vi "READ Falcon500 values.vi"(0 "PhoenixMotorControlDevRef":T1, 1 "refnum name":string, 3 "error in (no error)":errorcluster) -> (6 "PhoenixMotorControlDevRef 2":T1={"DeviceStatus"={"status"=FALSE, "code"=0, "source"=""}, "Type"=enum."PWM", "PWM"={"PWM Channel"=enum."Invalid", "DeadBand"={"Name"="", "maxPositivePwm"=0, "minPositivePwm"=0, "centerPwm"=0, "maxNegativePwm"=0, "minNegativePwm"=0, "angularRange"=0}}, "CAN"={"Device Number"=0, "SetOutput VI Ref"=variant(enum8{"Percent VBus", "Current", "Speed", "Position", "Voltage"} enum."Percent VBus"), "GetOutput VI Ref"=variant(refnum<k1> refnum), "Enable VI Ref"=variant(dbl 12.0), "Disable VI Ref"=variant(enum8{"Percent VBus", "Speed", "Position", "Slave", "Unchanged / Invalid", "Voltage Compensation", "Current", "Motion Profile"} enum."Percent VBus"), "Data"=variant}, "Invert"=FALSE, "DIO PWM"={"PWM \"Enable\" Channel"=enum."Invalid", "DIOChannel"=enum."Invalid", "PWM Rate"=0.0}}, 9 "error out":errorcluster)   [LabVIEW 2020]
uses:
  <vilib>/Rock Robotics/WPI/MotorControl/WPI_MotorControlDeviceRef.ctl
  <vilib>/Rock Robotics/WPI/MotorControl/WPI_MotorControlType.ctl
  <vilib>/Rock Robotics/SystemInterfaces/DIO/FPGA_DIOPWMChannel.ctl
  <vilib>/Rock Robotics/WPI/PWM/WPI_PWMDeadband.ctl
  <vilib>/Rock Robotics/SystemInterfaces/DIO/FPGA_DIOChannel.ctl
  <vilib>/Rock Robotics/WPI/ThirdParty/Phoenix-LabVIEW/Motor Controller/Get/CTRE_Phoenix_MotorController_GetVoltage.vi
  <vilib>/Rock Robotics/Network Tables/NT Write Number.vi
  <vilib>/Rock Robotics/WPI/ThirdParty/Phoenix-LabVIEW/Motor Controller/Get/CTRE_Phoenix_MotorController_GetSupplyAndStatorCurrent_Enhanced.vi
  <vilib>/Rock Robotics/WPI/ThirdParty/Phoenix-LabVIEW/Motor Controller/Get/CTRE_Phoenix_MotorController_GetSelectedSensorData.vi
  <vilib>/Rock Robotics/WPI/ThirdParty/Phoenix-LabVIEW/Motor Controller/Get/CTRE_Phoenix_MotorController_IntegratedSensorData_TalonFX.vi
  <vilib>/Rock Robotics/WPI/ThirdParty/Phoenix-LabVIEW/Motor Controller/Get/CTRE_Phoenix_MotorController_GetTemperature.vi
  <vilib>/Rock Robotics/WPI/ThirdParty/Phoenix-LabVIEW/Motor Controller/Get/CTRE_Phoenix_MotorController_GetLimitSwitchStates.vi
  <vilib>/Rock Robotics/Network Tables/NT Write Boolean.vi
panel:
  in  "ticks per rev":dbl=2048.0
  # "Note that the Falcon 500 encoder reports position as \"ticks\" of which there are 2048/rev and\nvelocity as ticks measured in a 100 ms period"
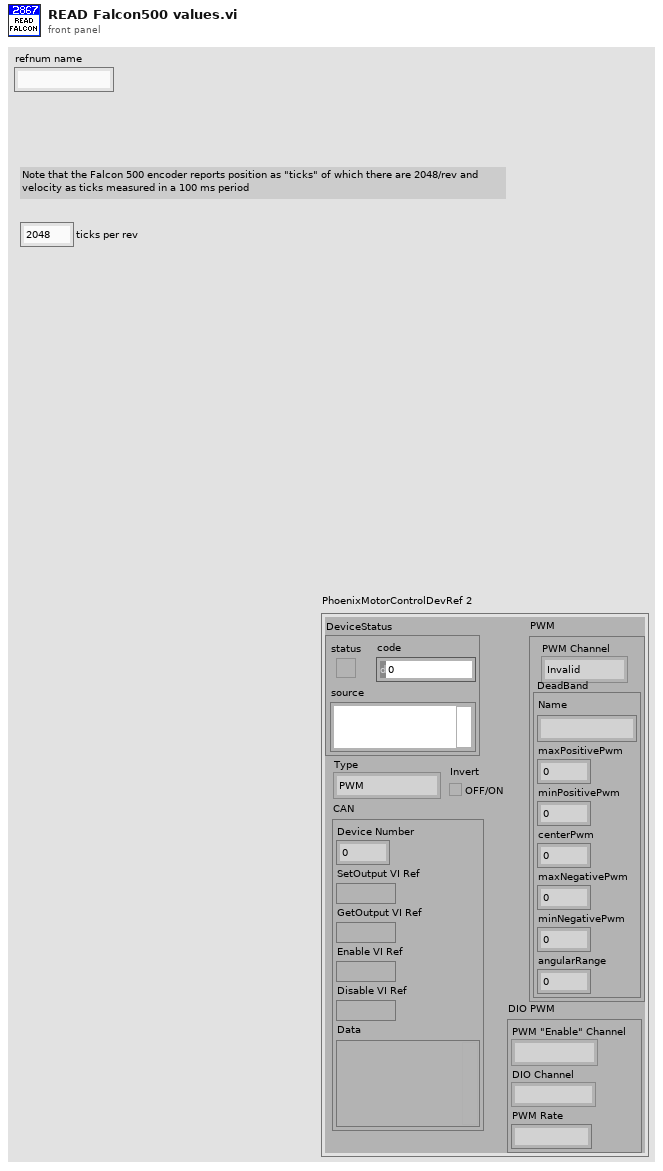
[diagram p1: front panel]
types:
  T1 = typedef "WPI_MotorControlDeviceRef.ctl" = cluster{"DeviceStatus":errorcluster, "Type":T2, "PWM":cluster{"PWM Channel":T3, "DeadBand":T4}, "CAN":cluster{"Device Number":u8, "SetOutput VI Ref":variant, "GetOutput VI Ref":variant, "Enable VI Ref":variant, "Disable VI Ref":variant, "Data":variant}, "Invert":bool, "DIO PWM":cluster{"PWM \"Enable\" Channel":T3, "DIOChannel":T5, "PWM Rate":dbl}}
  T2 = typedef "WPI_MotorControlType.ctl" = enum16{"PWM", "CAN", "DIO PWM"}
  T3 = typedef "FPGA_DIOPWMChannel.ctl" = enum8{"PWM 0", "PWM 1", "PWM 2", "PWM 3", "PWM 4", "PWM 5", "PWM 6", "PWM 7", "PWM 8", "PWM 9", "PWM MXP 0", "PWM MXP 1", "PWM MXP 2", "PWM MXP 3", "PWM MXP 4", "PWM MXP 5", "PWM MXP 6", "PWM MXP 7", "PWM MXP 8", "PWM MXP 9", "Invalid"}
  T4 = typedef "WPI_PWMDeadband.ctl" = cluster{"Name":string, "maxPositivePwm":i32, "minPositivePwm":i32, "centerPwm":i32, "maxNegativePwm":i32, "minNegativePwm":i32, "angularRange":u16}
  T5 = typedef "FPGA_DIOChannel.ctl" = enum8{"DIO 0", "DIO 1", "DIO 2", "DIO 3", "DIO 4", "DIO 5", "DIO 6", "DIO 7", "DIO 8", "DIO 9", "DIO MXP 0", "DIO MXP 1", "DIO MXP 2", "DIO MXP 3", "DIO MXP 4", "DIO MXP 5", "DIO MXP 6", "DIO MXP 7", "DIO MXP 8", "DIO MXP 9", "DIO MXP 10", "DIO MXP 11", "DIO MXP 12", "DIO MXP 13", "DIO MXP 14", "DIO MXP 15", "SPI Port CS1", "SPI Port CS2", "SPI Port CS3", "SPI Port MISO", "SPI Port MOSI", "Invalid"}
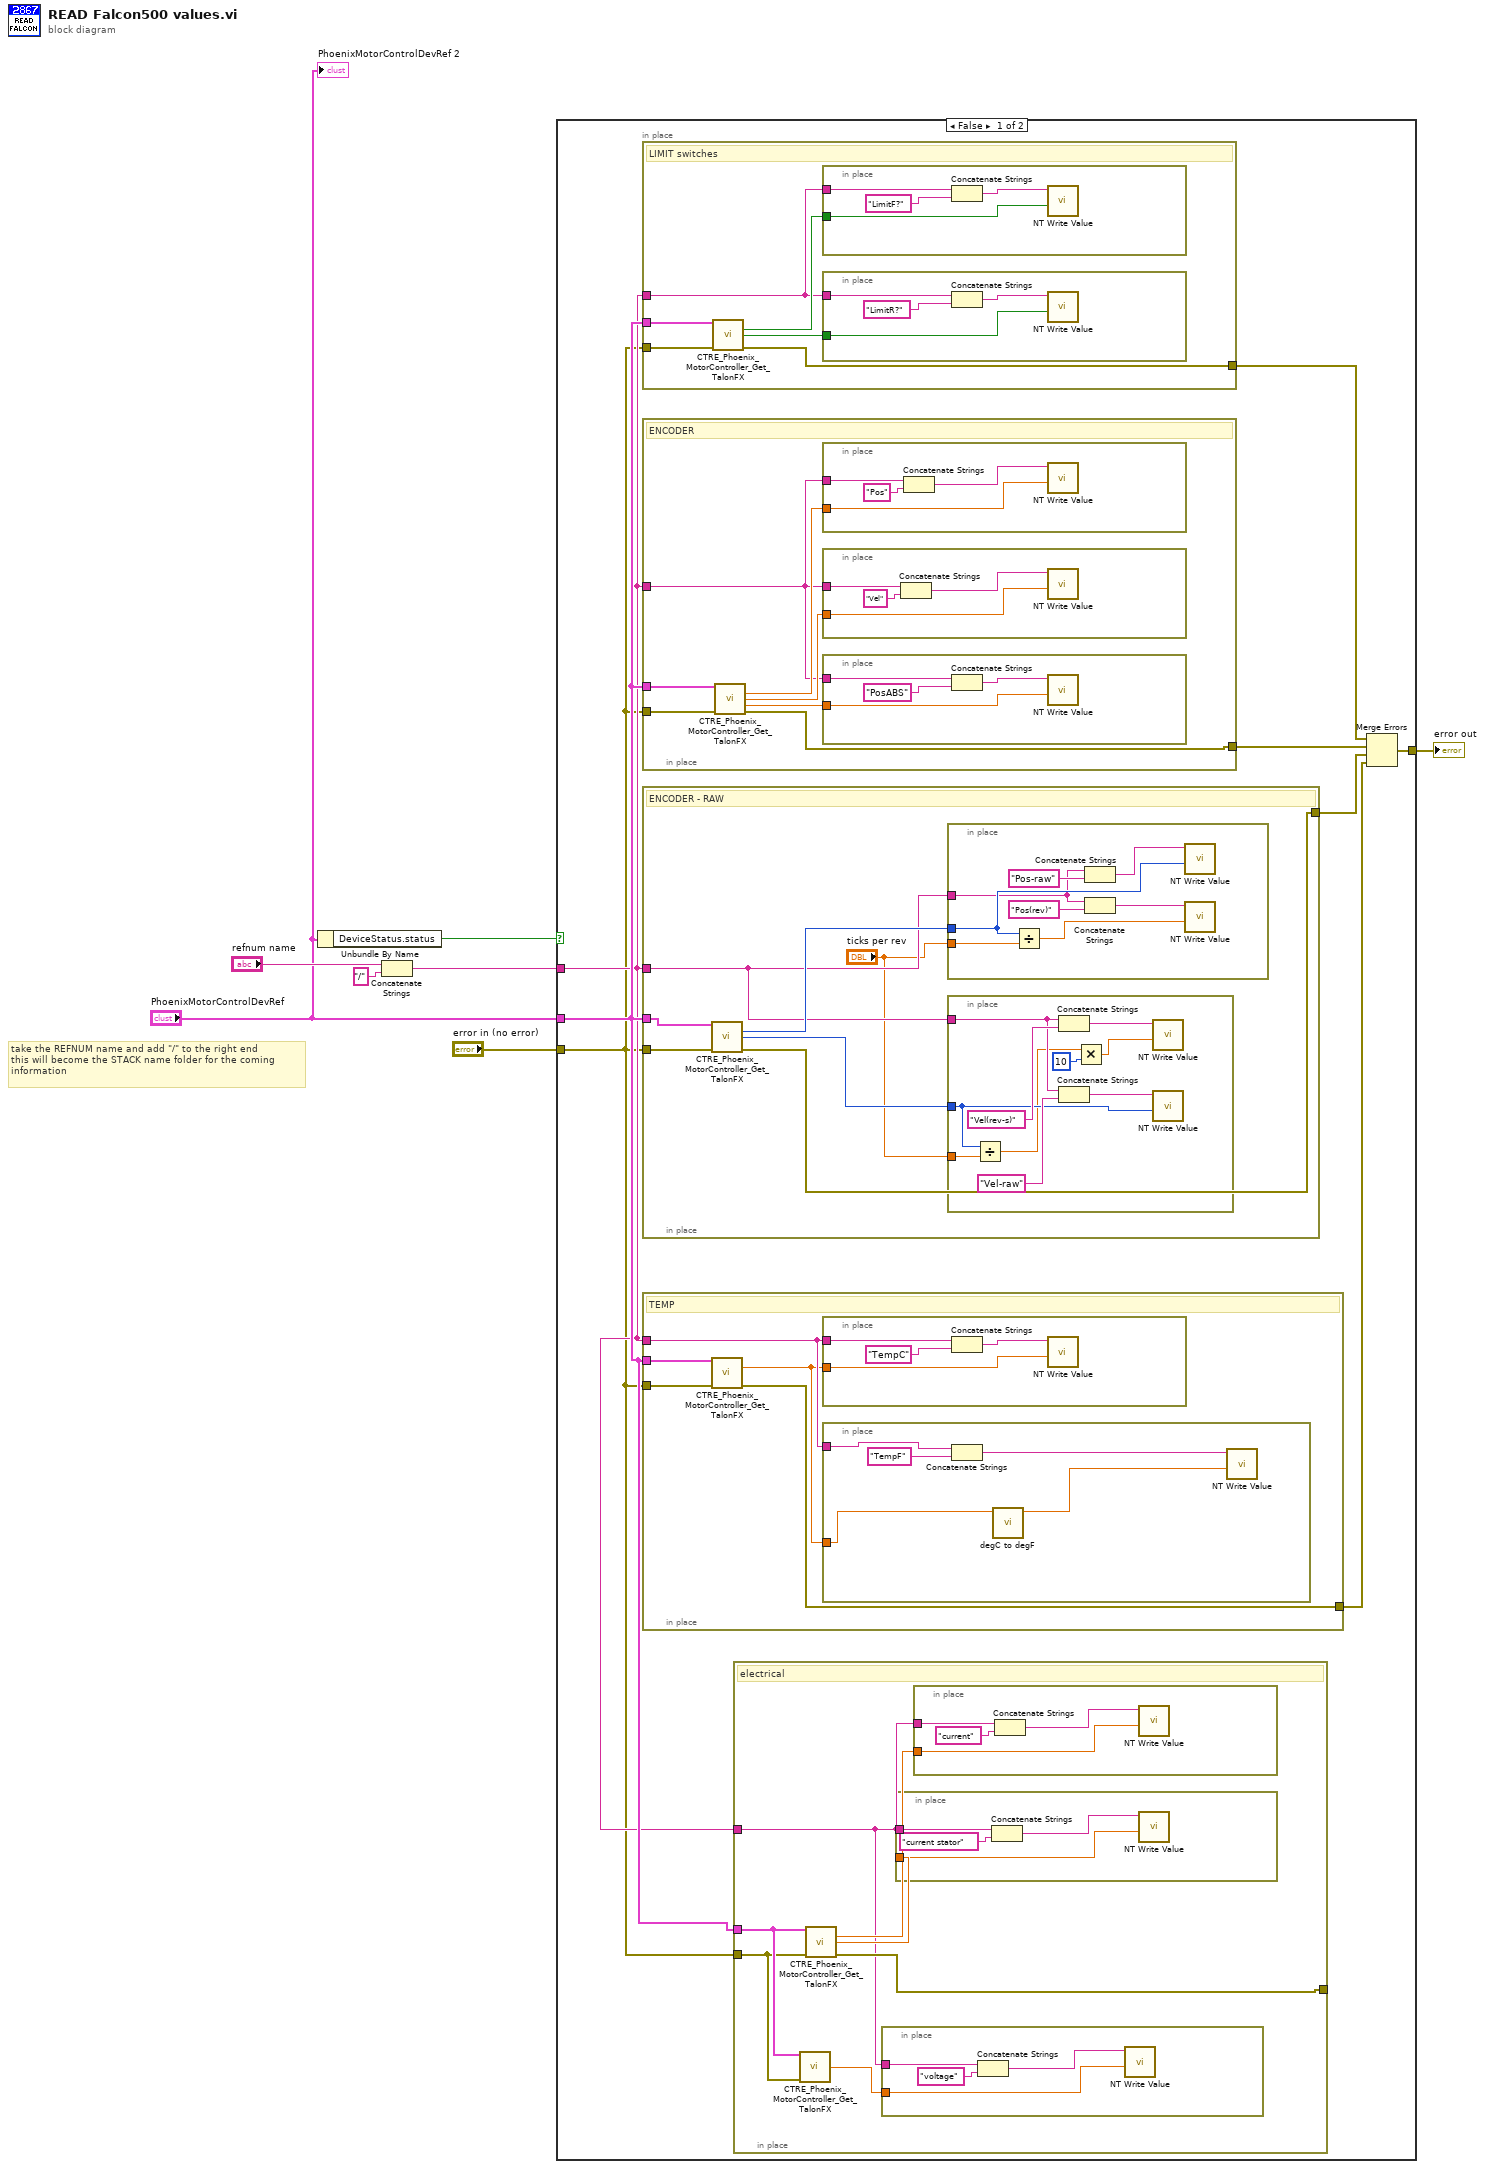
[diagram p0: block diagram]
diagram:
  # "take the REFNUM name and add \"/\" to the right end\nthis will become the STACK name folder for the coming\ninformation"
  n1 = Unbundle By Name("PhoenixMotorControlDevRef") -> ("DeviceStatus.status"=w2:bool)
  n2 = Concatenate Strings("refnum name", "/" ("string")) -> (w4:string)
  n3 = case shown="False" w2 {
    tunnel: "error in (no error)" -> [w8 _]
    tunnel: w4 -> [w9 _]
    tunnel: "PhoenixMotorControlDevRef" -> [w10 _]
    tunnel: [w15 _] -> w3
    frame False {
      n4 = in-place {
        in-place-border: w10 -> [w98]
        in-place-border: w8 -> [w97]
        in-place-border: [w94] -> w13
        in-place-border: w9 -> [w93]
        # "LIMIT switches"
        n5 = call-poly <vilib>:"CTRE_Phoenix_MotorController_Get_TalonFX.vi"("PhoenixMotorControlDevRef"=w98, "error in"=w97) -> ("Forward Limit Closed?"=w96:bool, "Reverse Limit Closed?"=w95:bool, "error out"=w94:errorcluster)  [unwired: 10 in, 1 out]
        n6 = in-place {
          in-place-border: w96 -> [w106]
          in-place-border: w93 -> [w105]
          n7 = Concatenate Strings(w105, "LimitF?" ("string")) -> (w104:string)
          n8 = call-poly <vilib>:"NT Write Value.vi"("Boolean"=w106, "Name"=w104) -> ()  [unwired: 9 in, 1 out]
        }
        n9 = in-place {
          in-place-border: w95 -> [w102]
          in-place-border: w93 -> [w101]
          n10 = Concatenate Strings(w101, "LimitR?" ("string")) -> (w100:string)
          n11 = call-poly <vilib>:"NT Write Value.vi"("Boolean"=w102, "Name"=w100) -> ()  [unwired: 9 in, 1 out]
        }
      }
      n12 = in-place {
        in-place-border: w10 -> [w80]
        in-place-border: [w76] -> w14
        in-place-border: w8 -> [w75]
        in-place-border: w9 -> [w74]
        # "ENCODER"
        n13 = call-poly <vilib>:"CTRE_Phoenix_MotorController_Get_TalonFX.vi"("PhoenixMotorControlDevRef"=w80, "error in"=w75) -> ("Position"=w79:dbl, "Velocity"=w78:dbl, "Absolute Position"=w77:dbl, "error out"=w76:errorcluster)  [unwired: 9 in, 1 out]
        n14 = in-place {
          in-place-border: w79 -> [w90]
          in-place-border: w74 -> [w89]
          n15 = Concatenate Strings(w89, "Pos" ("string")) -> (w92:string)
          n16 = call-poly <vilib>:"NT Write Value.vi"("Numeric"=w90, "Name"=w92) -> ()  [unwired: 9 in, 1 out]
        }
        n17 = in-place {
          in-place-border: w78 -> [w86]
          in-place-border: w74 -> [w85]
          n18 = Concatenate Strings(w85, "Vel" ("string")) -> (w88:string)
          n19 = call-poly <vilib>:"NT Write Value.vi"("Numeric"=w86, "Name"=w88) -> ()  [unwired: 9 in, 1 out]
        }
        n20 = in-place {
          in-place-border: w77 -> [w82]
          in-place-border: w74 -> [w81]
          n21 = Concatenate Strings(w81, "PosABS" ("string")) -> (w84:string)
          n22 = call-poly <vilib>:"NT Write Value.vi"("Numeric"=w82, "Name"=w84) -> ()  [unwired: 9 in, 1 out]
        }
      }
      n23 = in-place {
        in-place-border: w10 -> [w55]
        in-place-border: [w52] -> w12
        in-place-border: w8 -> [w51]
        in-place-border: w9 -> [w50]
        # "ENCODER - RAW"
        n24 = call-poly <vilib>:"CTRE_Phoenix_MotorController_Get_TalonFX.vi"("PhoenixMotorControlDevRef"=w55, "error in"=w51) -> ("Position (Raw Sensor Units)"=w54:i32, "Velocity (Raw Sensor Units per 100 ms)"=w53:i32, "error out"=w52:errorcluster)  [unwired: 10 in, 1 out]
        n25 = in-place {
          in-place-border: w54 -> [w71]
          in-place-border: w50 -> [w67]
          in-place-border: "ticks per rev" -> [w70]
          n26 = Divide(x=w71, y=w70) -> (x/y=w66:dbl)
          n27 = Concatenate Strings(w67, "Pos-raw" ("string")) -> (w73:string)
          n28 = Concatenate Strings(w67, "Pos(rev)" ("string")) -> (w68:string)
          n29 = call-poly <vilib>:"NT Write Value.vi"("Numeric"=w71, "Name"=w73) -> ()  [unwired: 9 in, 1 out]
          n30 = call-poly <vilib>:"NT Write Value.vi"("Numeric"=w66, "Name"=w68) -> ()  [unwired: 9 in, 1 out]
        }
        n31 = in-place {
          in-place-border: w53 -> [w58]
          in-place-border: w50 -> [w61]
          in-place-border: "ticks per rev" -> [w59]
          n32 = Divide(x=w58, y=w59) -> (x/y=w57:dbl)
          n33 = Concatenate Strings(w61, "Vel(rev-s)" ("string")) -> (w63:string)
          n34 = Concatenate Strings(w61, "Vel-raw" ("string")) -> (w65:string)
          n35 = Multiply(x=w57, y=10) -> (x*y=w56:dbl)
          n36 = call-poly <vilib>:"NT Write Value.vi"("Numeric"=w56, "Name"=w63) -> ()  [unwired: 9 in, 1 out]
          n37 = call-poly <vilib>:"NT Write Value.vi"("Numeric"=w58, "Name"=w65) -> ()  [unwired: 9 in, 1 out]
        }
      }
      n38 = in-place {
        in-place-border: w10 -> [w39]
        in-place-border: [w38] -> w11
        in-place-border: w8 -> [w37]
        in-place-border: w9 -> [w36]
        # "TEMP"
        n39 = call-poly <vilib>:"CTRE_Phoenix_MotorController_Get_TalonFX.vi"("PhoenixMotorControlDevRef"=w39, "error in"=w37) -> ("Temperature (C)"=w35:dbl, "error out"=w38:errorcluster)  [unwired: 11 in, 1 out]
        n40 = in-place {
          in-place-border: w35 -> [w46]
          in-place-border: w36 -> [w45]
          n41 = Concatenate Strings(w45, "TempC" ("string")) -> (w48:string)
          n42 = call-poly <vilib>:"NT Write Value.vi"("Numeric"=w46, "Name"=w48) -> ()  [unwired: 9 in, 1 out]
        }
        n43 = in-place {
          in-place-border: w36 -> [w42]
          in-place-border: w35 -> [w41]
          n44 = Concatenate Strings(w42, "TempF" ("string")) -> (w44:string)
          n45 = call "degC to degF.vi"("degreesC"=w41) -> ("degreesF"=w40:dbl)  [unwired: 10 in]
          n46 = call-poly <vilib>:"NT Write Value.vi"("Numeric"=w40, "Name"=w44) -> ()  [unwired: 9 in, 1 out]
        }
      }
      n47 = in-place {
        in-place-border: w10 -> [w18]
        in-place-border: [w20] -> _
        in-place-border: w8 -> [w17]
        in-place-border: w9 -> [w19]
        # "electrical"
        n48 = call-poly <vilib>:"CTRE_Phoenix_MotorController_Get_TalonFX.vi"("PhoenixMotorControlDevRef"=w18, "error in"=w17) -> ("Output Voltage"=w16:dbl)  [unwired: 9 in, 4 out]
        n49 = call-poly <vilib>:"CTRE_Phoenix_MotorController_Get_TalonFX.vi"("PhoenixMotorControlDevRef"=w18, "error in"=w17) -> ("Supply Current"=w22:dbl, "Stator Current"=w21:dbl, "error out"=w20:errorcluster)  [unwired: 10 in, 1 out]
        n50 = in-place {
          in-place-border: w16 -> [w24]
          in-place-border: w19 -> [w23]
          n51 = Concatenate Strings(w23, "voltage" ("string")) -> (w26:string)
          n52 = call-poly <vilib>:"NT Write Value.vi"("Numeric"=w24, "Name"=w26) -> ()  [unwired: 9 in, 1 out]
        }
        n53 = in-place {
          in-place-border: w21 -> [w28]
          in-place-border: w19 -> [w27]
          n54 = Concatenate Strings(w27, "current stator" ("string")) -> (w30:string)
          n55 = call-poly <vilib>:"NT Write Value.vi"("Numeric"=w28, "Name"=w30) -> ()  [unwired: 9 in, 1 out]
        }
        n56 = in-place {
          in-place-border: w22 -> [w32]
          in-place-border: w19 -> [w31]
          n57 = Concatenate Strings(w31, "current" ("string")) -> (w34:string)
          n58 = call-poly <vilib>:"NT Write Value.vi"("Numeric"=w32, "Name"=w34) -> ()  [unwired: 9 in, 1 out]
        }
      }
      n59 = Merge Errors(w13, w14, w12, w11) -> (w15:errorcluster)
    }
    frame True {
    }
  }
  "error out" <- w3
  "PhoenixMotorControlDevRef 2" <- "PhoenixMotorControlDevRef"
